vi "OA_Col-SetData.vi"(0 "Origin.Column":refnum<k7>, 3 "error in (no error)":errorcluster, 4 "data":variant, 8 "nOffset":i32) -> (6 "Origin.Column Out":refnum<k7>, 7 "SetData":bool, 9 "error out":errorcluster)   [LabVIEW 2012]
doc: "Put a numeric array into a Column"
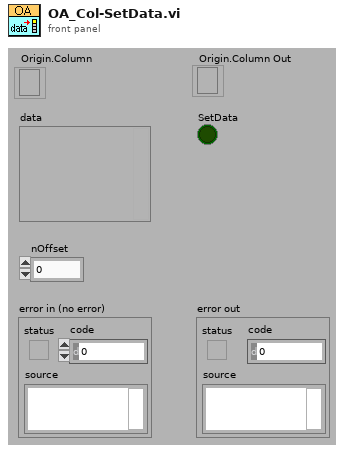
[diagram p1: front panel]
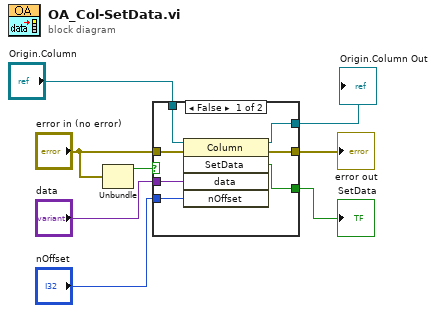
[diagram p0: block diagram]
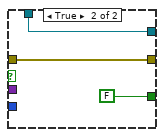
[diagram p2: hidden frame]
diagram:
  n1 = Unbundle("error in (no error)") -> ("status"=w3:bool)  [unwired: 2 out]
  n2 = case shown="False" w3 {
    tunnel: "error in (no error)" -> [w14 w18]
    tunnel: "data" -> [w12 _]
    tunnel: "nOffset" -> [w13 _]
    tunnel: [w9 w16] -> w1
    tunnel: [w10 w18] -> w6
    tunnel: [w11 FALSE ("SetData")] -> w5
    tunnel: "Origin.Column" -> [w15 w16]
    frame False {
      n3 = invoke class="Column" method="SetData"(reference=w15, error in=w14, "data"=w12, "nOffset"=w13) -> (reference out=w9:refnum<k7>, error out=w10:errorcluster, "SetData"=w11:bool)  [unwired: 1 in, 2 out]
    }
    frame True {
    }
  }
  "error out" <- w6
  "SetData" <- w5
  "Origin.Column Out" <- w1
